vi "Connect Standalone Wlan Card.vi"(7 "DutNum":i32, 8 "error in (no error)":errorcluster, 9 "ErrMsg":string, 10 "dllPath":string, 11 "USER_DUT_IP":string) -> (0 "error out":errorcluster, 1 "ErrMsg out":string, 2 "dllPath out":string, 3 "function return":u32, 4 "USER_DUT_IP out":string, 5 "Connect ?":bool)   [LabVIEW 2013, in "QCAWLAN_DLL.lvlib"]
doc: "QCA_DLL_Export HANDLE ConnectStandaloneWlanCard(char* USER_DUT_IP, char* dllPath, char* ErrMsg, int DutNum);"
uses:
  QCAWLAN_DLL.lvlib
  QCAWLAN_DLL.dll
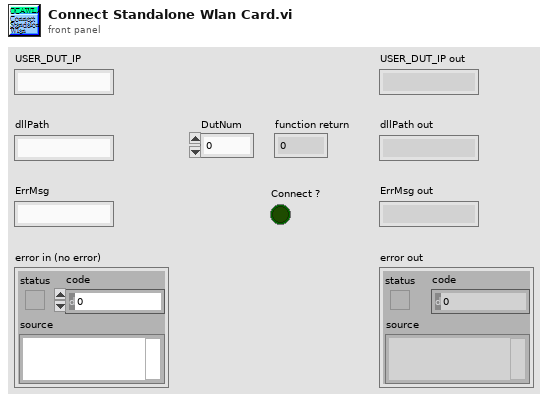
[diagram p1: front panel]
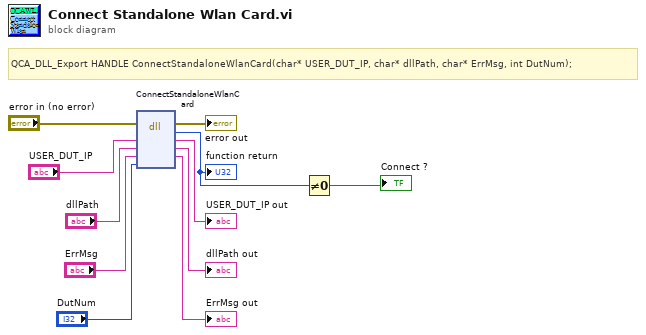
[diagram p0: block diagram]
diagram:
  # "QCA_DLL_Export HANDLE ConnectStandaloneWlanCard(char* USER_DUT_IP, char* dllPath, char* ErrMsg, int DutNum);"
  n1 = dll-call lib="C:/Connectivity Client - MIMO/PlugIn/QCAWLAN_DLL.*" fn="ConnectStandaloneWlanCard"(error in="error in (no error)", "USER_DUT_IP"="USER_DUT_IP", "dllPath"="dllPath", "ErrMsg"="ErrMsg", "DutNum"="DutNum") -> (error out=→"error out":errorcluster, w2:u32, "USER_DUT_IP"=→"USER_DUT_IP out":string, "dllPath"=→"dllPath out":string, "ErrMsg"=→"ErrMsg out":string)  [unwired: 3 in, 1 out]
  "function return" <- w2
  n2 = Not Equal To 0?(x=w2) -> (x != 0?=→"Connect ?":bool)
